vi "create reference.vi"(7 "project name":string, 8 "error in":errorcluster, 11 "queue in":refnum<queue>) -> (0 "error out":errorcluster, 3 "dvr ref":refnum<data-value>)   [LabVIEW 2023, in "Publisher Subscriber.lvlib"]
uses:
  <userlib>/_Publisher Subscriber/Publisher Subscriber.lvlib
  <userlib>/_Publisher Subscriber/Controls/data cluster.ctl
  <userlib>/_Publisher Subscriber/Controls/node dvr data.ctl
  <userlib>/_Publisher Subscriber/Controls/subscription bank ref.ctl
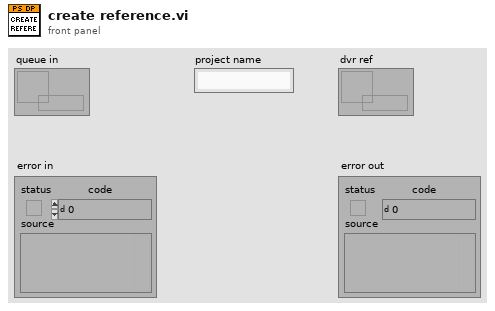
[diagram p1: front panel]
types:
  T1 = cluster{"subscription map ref":refnum<data-value>, "variable dvr refs":refnum<data-value>}
  T2 = typedef "Publisher Subscriber.lvlib/node dvr data.ctl" = cluster{"queue ref":refnum<queue>, "Subscription Bank Ref":refnum<data-value>, "Command":string, "Data":variant, "Subscriptions []":set{string}, "Variables DVR Ref":refnum<data-value>}
  T3 = typedef "Publisher Subscriber.lvlib/subscription bank ref.ctl" = map{string, set{refnum<queue>}}
  T4 = cluster{"data value reference":refnum<data-value>, "data value reference":refnum<data-value>}
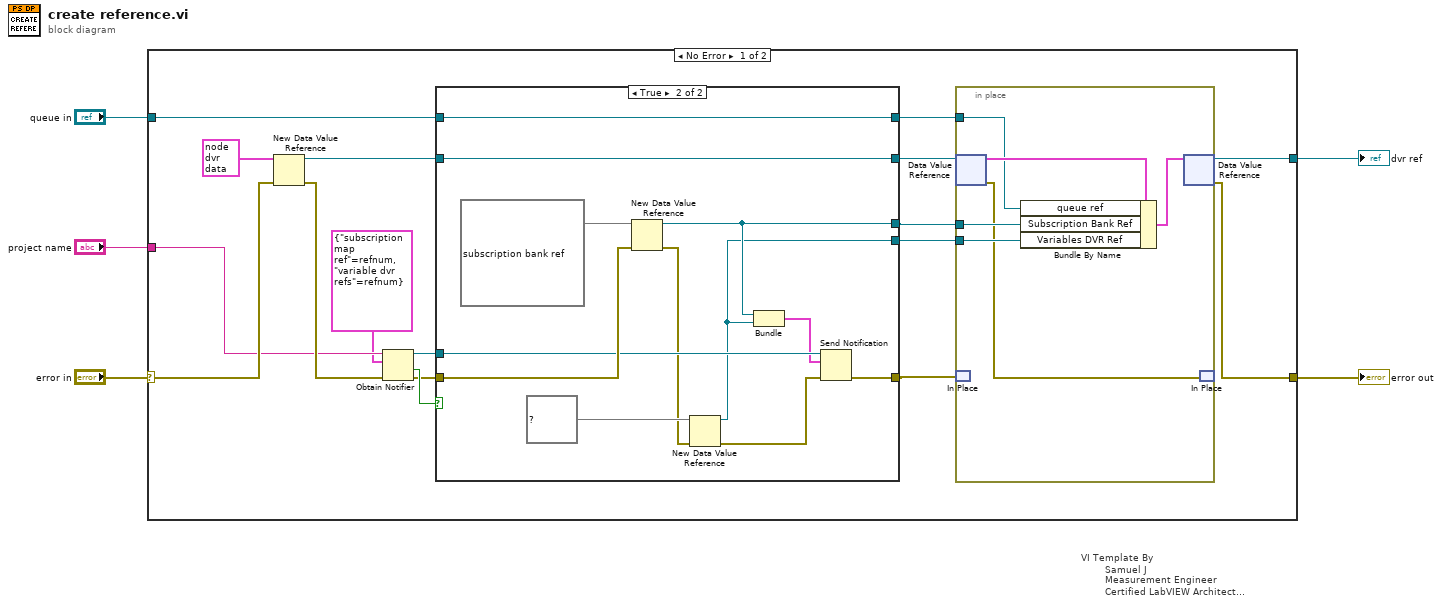
[diagram p0: block diagram]
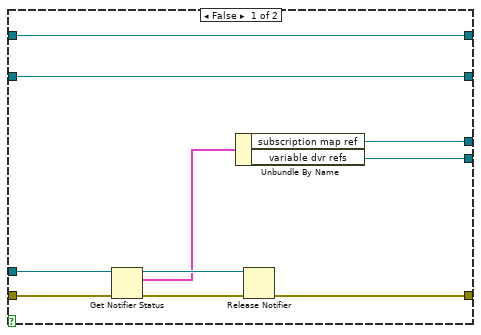
[diagram p2: hidden frame]
diagram:
  n1 = case "VI Template By\n        Samuel J\n        Measurement Engineer\n        Certified LabVIEW Architect\n        Vestas Technology R&D Chennai" shown="No Error" "error in" {
    selector: "error in" -> [w18 w51]
    tunnel: [w6 w51] -> w4
    tunnel: "project name" -> [w12 _]
    tunnel: "queue in" -> [w13 _]
    tunnel: [w7 _] -> w1
    frame No Error {
      n2 = New Data Value Reference(data value=T2 {"queue ref"=refnum, "Subscription Bank Ref"=refnum, "Command"="", "Data"=variant, "Subscriptions []"={}, "Variables DVR Ref"=refnum} ("Cluster"), error in=w18) -> (data value reference=w16:refnum<data-value>, error out=w17:errorcluster)
      n3 = Obtain Notifier(name (unnamed)=w12, notification data type=T1 {"subscription map ref"=refnum, "variable dvr refs"=refnum} ("Cluster"), error in (no error)=w17) -> (notifier out=w19:refnum<notifier>, created new?=w21:bool, error out=w20:errorcluster)  [unwired: 1 in]
      n4 = case shown="True" w21 {
        tunnel: w20 -> [w38 w50]
        tunnel: w19 -> [w37 w45]
        tunnel: [w30 w43] -> w10
        tunnel: [w34 w49] -> w11
        tunnel: w16 -> [w33 w48]
        tunnel: [w33 w48] -> w15
        tunnel: [w32 w47] -> w14
        tunnel: w13 -> [w32 w47]
        tunnel: [w29 w41] -> w8
        frame False {
          n5 = Get Notifier Status(notifier=w37, error in (no error)=w38) -> (notifier out=w36:refnum<notifier>, current notification=w31:T1, error out=w35:errorcluster)  [unwired: 2 out]
          n6 = Unbundle By Name(w31) -> ("subscription map ref"=w30:refnum<data-value>, "variable dvr refs"=w29:refnum<data-value>)
          n7 = Release Notifier(notifier=w36, error in (no error)=w35) -> (error out=w34:errorcluster)  [unwired: 1 in, 2 out]
        }
        frame True {
          n8 = New Data Value Reference(data value=T3 {} ("Map"), error in=w50) -> (data value reference=w43:refnum<data-value>, error out=w40:errorcluster)
          n9 = New Data Value Reference(data value=map{string, variant} {} ("global map"), error in=w40) -> (data value reference=w41:refnum<data-value>, error out=w39:errorcluster)
          n10 = Bundle("data value reference"=w43, "data value reference"=w41) -> (w42:T4)  [unwired: 1 in]
          n11 = Send Notification(notification=w42, notifier=w45, error in (no error)=w39) -> (error out=w49:errorcluster)  [unwired: 1 out]
        }
      }
      n12 = in-place {
        in-place-border: w14 -> [w26]
        in-place-border: w10 -> [w25]
        in-place-border: w8 -> [w24]
        n13 = in-place-dvr #1(w15) -> (w28:T2, w23:errorcluster)
        n14 = in-place-match #2(w11) -> ()  [unwired: 1 out]
        n15 = Bundle By Name(cluster=w28, "queue ref"=w26, "Subscription Bank Ref"=w25, "Variables DVR Ref"=w24) -> (w27:T2)
        n16 = in-place-dvr #1(w27) -> (w7:refnum<data-value>, w6:errorcluster)
        n17 = in-place-match #2(w23) -> ()  [unwired: 1 out]
      }
    }
    frame Error {
    }
  }
  "error out" <- w4
  "dvr ref" <- w1
